vi "Looding_file.vi"(8 "error in":errorcluster, 10 "组合框":string(combo), 11 "仪器通讯端口":refnum<visa-resource-name>) -> (0 "错误输出":errorcluster, 3 "VISA资源名称输出":refnum<visa-resource-name>)   [LabVIEW 2018]
panel:
  out "连接的字符串":string
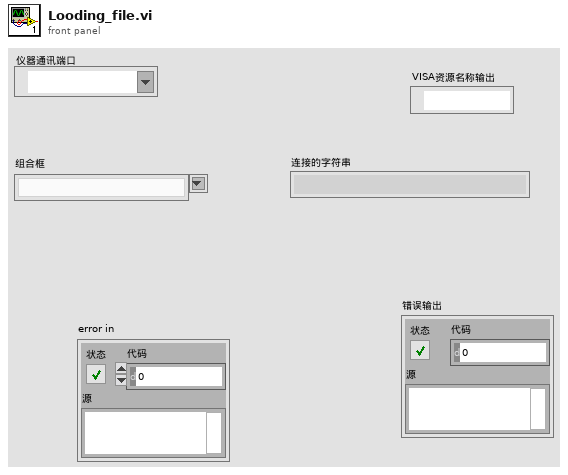
[diagram p1: front panel]
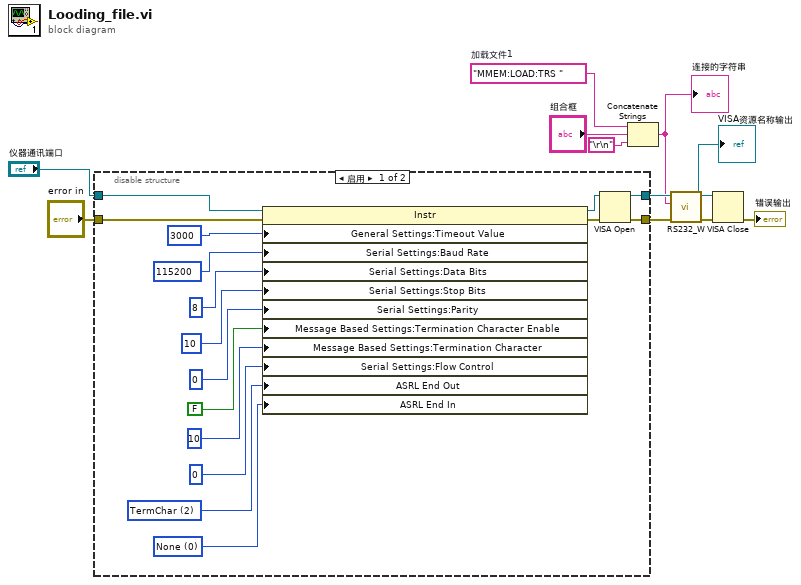
[diagram p0: block diagram]
diagram:
  w3 = "MMEM:LOAD:TRS "  # 加载文件1
  n1 = disable-structure shown="启用" {
    disable-tunnel: [w27 w28] -> w10
    disable-tunnel: [w26 _] -> w11
    disable-tunnel: "仪器通讯端口" -> [w23 w28]
    disable-tunnel: "error in" -> [w12 _]
    frame Enabled {
      w17 = u16 0 items=["None", "Last Bit", "TermChar"] ("Serial Settings:End Mode for Reads")
      w19 = u16 2 items=["None", "Last Bit", "TermChar", "Break"] ("Serial Settings:End Mode for Writes")
      n2 = property class="Instr"(reference=w23, error in=w12, "General Settings:Timeout Value"=u32 3000, "Serial Settings:Baud Rate"=u32 115200, "Serial Settings:Data Bits"=u16 8, "Serial Settings:Stop Bits"=u16 10, "Serial Settings:Parity"=u16 0, "Message Based Settings:Termination Character Enable"=FALSE ("TermChar En"), "Message Based Settings:Termination Character"=u8 10, "Serial Settings:Flow Control"=u16 0, "ASRL End Out"=w19, "ASRL End In"=w17) -> (reference out=w24:refnum<visa-resource-name>, error out=w25:errorcluster)
      n3 = VISA Open ("VISA打开")(error in (no error)=w25, VISA resource name=w24) -> (VISA resource name=w27:refnum<visa-resource-name>, error out=w26:errorcluster)  [unwired: 3 in]
    }
    frame Disabled {
    }
  }
  n4 = Concatenate Strings(w3, "组合框", "\r\n") -> (w1:string)
  "连接的字符串" <- w1
  n5 = call "RS232_W.vi"("error in (no error)"=w11, "CMD"=w1, "VISA资源名称"=w10) -> ("error out"=w7:errorcluster, "VISA资源名称输出"=w6:refnum<visa-resource-name>)  [unwired: 6 in, 1 out]
  "VISA资源名称输出" <- w6
  n6 = VISA Close(VISA resource name=w6, error in (no error)=w7) -> (error out=→"错误输出":errorcluster)
